vi "ep_Peak Values and Crest Factor.vi"(8 "error in (no error)":errorcluster, 10 "RMS":dbl[](array[numeric]) format="%.2p", 11 "data":waveform(dbl)[](array[waveform])) -> (0 "error out":errorcluster, 1 "crest factor":dbl[](array[numeric]), 2 "- peak values":dbl[](array[numeric]), 3 "+peak values":dbl[](array[numeric]))   [LabVIEW 2024]
doc: "Calculates the peak values and crest factor of input signals."
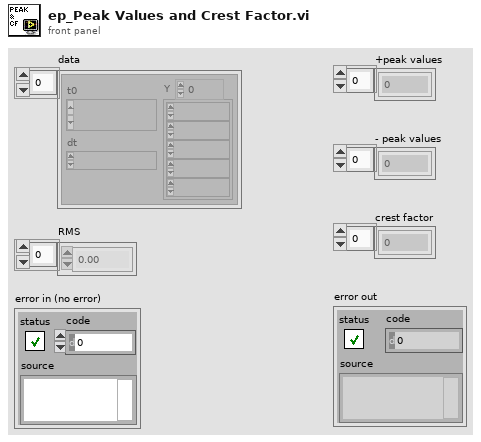
[diagram p1: front panel]
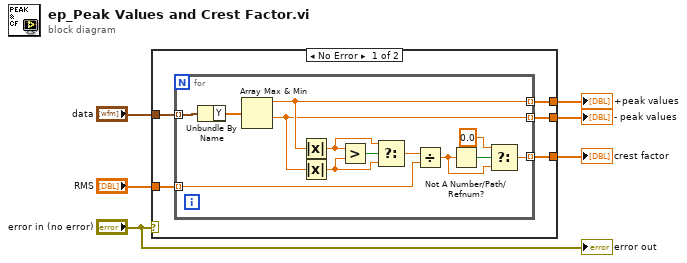
[diagram p0: block diagram]
diagram:
  n1 = case shown="No Error" "error in (no error)" {
    tunnel: "data" -> [w11 _]
    tunnel: "RMS" -> [w10 _]
    tunnel: [w9 _] -> w1
    tunnel: [w8 _] -> w2
    tunnel: [w7 _] -> w3
    frame No Error {
      n2 = for {
        tunnel: w11 -> [w24] mode=indexing
        tunnel: [w22] -> w7 mode=indexing
        tunnel: [w21] -> w8 mode=indexing
        tunnel: w10 -> [w16] mode=indexing
        tunnel: [w12] -> w9 mode=indexing
        n3 = Unbundle By Name(w24) -> ("Y"=w23:dbl[])
        n4 = Array Max & Min(array=w23) -> (max value=w22:dbl, min value=w21:dbl)  [unwired: 2 out]
        n5 = Absolute Value(x=w22) -> (abs(x)=w18:dbl)
        n6 = Absolute Value(x=w21) -> (abs(x)=w19:dbl)
        n7 = Greater?(x=w18, y=w19) -> (0:w20:bool)
        n8 = Select(t=w18, s=w20, f=w19) -> (s? t:f=w17:dbl)
        n9 = Divide(x=w17, y=w16) -> (x/y=w13:dbl)
        n10 = Not A Number/Path/Refnum?(number/path/refnum=w13) -> (NaN/Path/Refnum?=w15:bool)
        n11 = Select(t=0.0, s=w15, f=w13) -> (s? t:f=w12:dbl)
      }
    }
    frame Error {
    }
  }
  "+peak values" <- w3
  "- peak values" <- w2
  "crest factor" <- w1
  "error out" <- "error in (no error)"
